vi "Handle Command.vi"(8 "error in":errorcluster, 10 "Change Speaker State in":refnum<class "Change Speaker State.lvclass">, 11 "Object In":refnum<class>) -> (0 "error out":errorcluster, 1 "Command Successful?":bool, 2 "Change Speaker State out":refnum<class "Change Speaker State.lvclass">, 3 "Object Out":refnum<class>)   [LabVIEW 2014, in "ePAS Library.lvlib" / "Change Speaker State.lvclass"]
doc: "Change the current speaker position, log that position if the command is good (record the error if it is not) and update the data object."
uses:
  Change Speaker State.lvclass
  FPGA/Session/Exscalabar FPGA.lvclass
  Instrument/ePAS.lvclass
  reusable/PAS/Data/Main/PAS Data.lvclass
  Instrument/ePAS.lvclass/ePAS.ctl
  reusable/Instrument/Instrument.lvclass/Instrument.ctl
  Change Speaker State.lvclass/Change Speaker State.ctl
  FPGA/Session/Exscalabar FPGA.lvclass/Exscalabar FPGA.ctl
  Instrument/Accessors/Read FPGA Session.vi
  reusable/Instrument/Read Data.vi
  reusable/Instrument/Read Log Session.vi
  FPGA/Session/Read Ex FPGA Ref.vi
  reusable/Instrument/Write Data.vi
  reusable/Instrument/Read ExtCom.vi
  reusable/PAS/Main/Read Switch Ref.vi
  <vilib>/Utility/error.llb/Error Cluster From Error Code.vi
  <vilib>/rvi/errors/niLvFpgaAdjustHostInterfaceError.vi
  reusable/PAS/Data/Main/Write drive.vi
  reusable/PAS/Main/Set Speaker Switch.vi
  reusable/PAS/Main/Write Speaker Reference.vi
  <vilib>/DAQmx/write.llb/DAQmx Write (Digital Bool 1Line 1Point).vi
  <userlib>/_Session Fwk/Session - Root.lvclass
  reusable/Data/Data.lvclass
  reusable/Switch/Switch.lvclass
  FPGA/R FPGA Ref.ctl
  <vilib>/rvi/interface/nirviReadWriteControl/nirviReadWriteControl.xnode
  FPGA Bitfiles/FPGAServerV2.lvbitx
  reusable/Session APIs/Session Log/System Log.lvclass
  ePAS Library.lvlib
  NiFpgaLv.dll
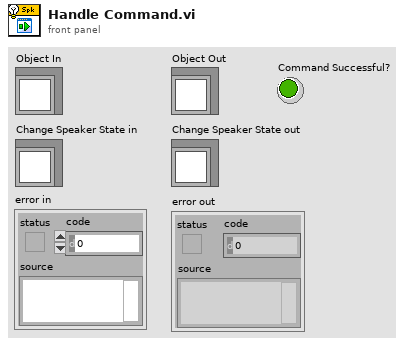
[diagram p1: front panel]
types:
  T1 = typedef "Session - Root.lvclass/Session Handle.ctl" = refnum<data-value>
  T2 = typedef "ePAS Library.lvlib/R FPGA Ref.ctl" = refnum<k20>
  T3 = cluster{"State":bool, "State":bool, "State":bool, "State":bool, "State":bool}
  T4 = cluster{"tag":string, "section":string, "data":variant}
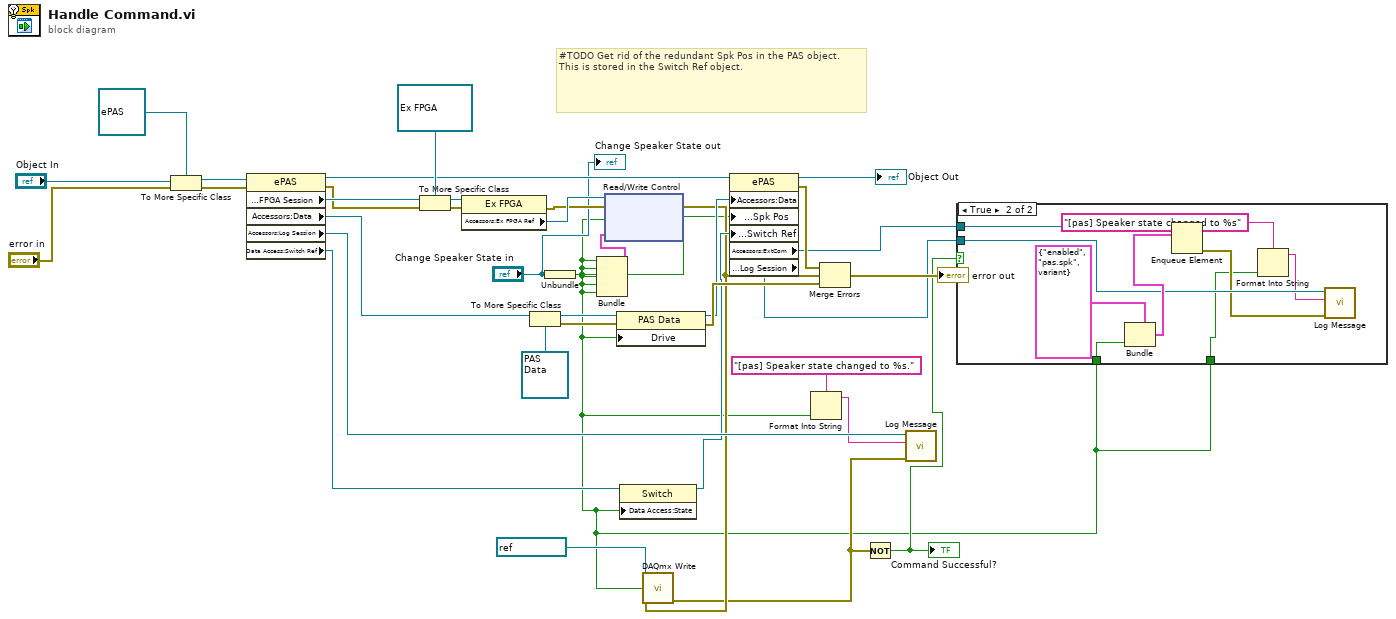
[diagram p0: block diagram]
diagram:
  # "#TODO Get rid of the redundant Spk Pos in the PAS object.  This is stored in the Switch Ref object."
  n1 = To More Specific Class(target class=refnum<class "ePAS.lvclass"> refnum ("ePAS.lvclass"), reference="Object In", error in="error in") -> (specific class reference=w32:refnum<class "ePAS.lvclass">, error out=w31:errorcluster)
  n2 = property class="ePAS"(reference=w32, error in=w31) -> (reference out=w17:refnum<class "ePAS.lvclass">, error out=w20:errorcluster, "Accessors:FPGA Session"=w29:T1, "Accessors:Data"=w28:refnum<class "Data.lvclass">, "Accessors:Log Session"=w24:T1, "Data Access:Switch Ref"=w14:refnum<class "Switch.lvclass">)
  n3 = To More Specific Class(target class=refnum<data-value> refnum ("Session Handle"), reference=w29, error in=w20) -> (specific class reference=w35:refnum<data-value>, error out=w34:errorcluster)
  n4 = property class="Ex FPGA"(reference=w35, error in=w34) -> (error out=w21:errorcluster, "Accessors:Ex FPGA Ref"=w26:T2)  [unwired: 1 out]
  n5 = To More Specific Class(target class=refnum<class "PAS Data.lvclass"> refnum ("PAS Data"), reference=w28) -> (specific class reference=w25:refnum<class "PAS Data.lvclass">, error out=w19:errorcluster)  [unwired: 1 in]
  n6 = Unbundle("Change Speaker State in") -> (w2:bool)
  n7 = Bundle("State"=w2, "State"=w2, "State"=w2, "State"=w2, "State"=w2) -> (w1:T3)  [unwired: 1 in]
  n8 = xnode "Read/Write Control"("FPGA VI Reference In"=w26, "error in"=w21, "Spk Enable"=w2, "iSpk Enable"=w1) -> ("error out"=w7:errorcluster)  [unwired: 1 out]
  n9 = property class="PAS Data"(reference=w25, error in=w19, "Drive"=w2) -> (reference out=w16:refnum<class "PAS Data.lvclass">, error out=w18:errorcluster)
  n10 = property class="Switch"(reference=w14, "Data Access:State"=w2) -> (reference out=w13:refnum<class "Switch.lvclass">)  [unwired: 1 in, 1 out]
  n11 = call-poly <vilib>:"DAQmx Write.vi"("task/channels in"=refnum<k21> "Spk LED", "data"=w2, "error in"=w7) -> ("error out"=w6:errorcluster)  [unwired: 10 in, 2 out]
  n12 = property class="ePAS"(reference=w17, "Accessors:Data"=w16, "Data Access:Spk Pos"=w2, "Data Access:Switch Ref"=w13) -> (reference out=→"Object Out":refnum<class "ePAS.lvclass">, error out=w15:errorcluster, "Accessors:ExtCom"=w4:refnum<queue>, "Accessors:Log Session"=w3:T1)  [unwired: 1 in]
  n13 = Format Into String(format string="[pas] Speaker state changed to %s.", w2) -> (resulting string=w22:string)  [unwired: 2 in, 1 out]
  n14 = Merge Errors(w15, w7, w18) -> (→"error out":errorcluster)
  n15 = Not(x=w6) -> (.not. x?=w5:bool)
  "Command Successful?" <- w5
  n16 = call "Log Message.vi"("error in"=w6, "MSG In"=w22, "session in"=w24) -> ()  [unwired: 7 in, 2 out]
  n17 = case shown="True" w5 {
    tunnel: w4 -> [_ w45]
    tunnel: w2 -> [_ w40]
    tunnel: w3 -> [_ w42]
    tunnel: w2 -> [_ w37]
    frame False {
    }
    frame True {
      n18 = Bundle(cluster=T4 {"tag"="enabled", "section"="pas.spk", "data"=variant} ("element"), "data"=w40) -> (w43:T4)  [unwired: 2 in]
      n19 = Enqueue Element(queue=w45, element=w43) -> (error out=w38:errorcluster)  [unwired: 2 in, 2 out]
      n20 = Format Into String(format string="[pas] Speaker state changed to %s", w37) -> (resulting string=w39:string)  [unwired: 2 in, 1 out]
      n21 = call "Log Message.vi"("error in"=w38, "MSG In"=w39, "session in"=w42) -> ()  [unwired: 7 in, 2 out]
    }
  }
  "Change Speaker State out" <- "Change Speaker State in"
